vi "SMTP Email Convert SJIS to JIS.vi"(11 "text in":string) -> (3 "text out":string)   [LabVIEW 2012, in "NewNI_SMTPEmail.lvlib"]
doc: "This VI converts SJIS input code to JIS."
uses:
  NewNI_SMTPEmail.lvlib
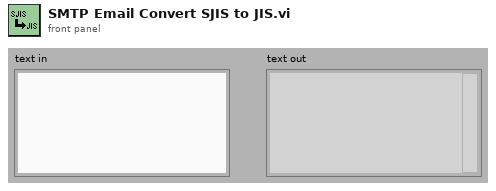
[diagram p1: front panel]
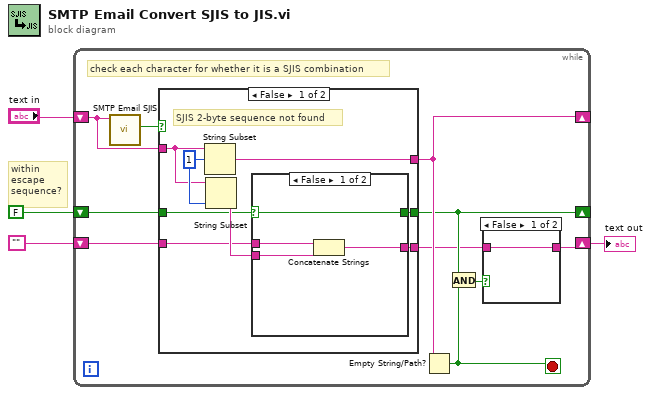
[diagram p0: block diagram]
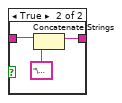
[diagram p2: hidden frame]
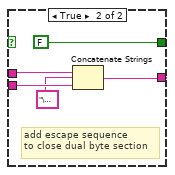
[diagram p3: hidden frame]
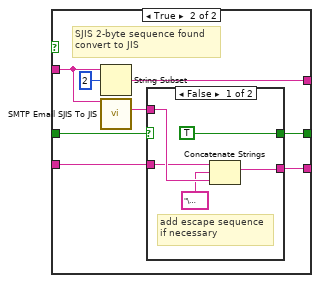
[diagram p4: hidden frame]
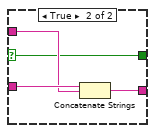
[diagram p5: hidden frame]
diagram:
  # "within\nescape\nsequence?"
  n1 = while {
    shift-right: [w10] -> _
    shift-left: "text in" -> [w13]
    shift-right: [w5] -> w1
    shift-left: "" -> [w12]
    shift-right: [w9] -> _
    shift-left: FALSE -> [w11]
    stop <- w8 stop-if-true
    # "check each character for whether it is a SJIS combination"
    n2 = call "SMTP Email SJIS.vi"("text"=w13) -> ("isSJIS?"=w14:bool)  [unwired: 10 out]
    n3 = case shown="False" w14 {
      tunnel: w13 -> [w24 w39]
      tunnel: [w23 w42] -> w10
      tunnel: w12 -> [w22 w41]
      tunnel: [w20 w40] -> w6
      tunnel: w11 -> [w21 w37]
      tunnel: [w19 w36] -> w9
      frame False {
        w26 = 1 ("offset (0)")
        # "SJIS 2-byte sequence not found"
        n4 = String Subset(string=w24, offset (0)=w26) -> (substring=w23:string)  [unwired: 1 out]
        n5 = String Subset(string=w24, length (rest)=w26) -> (substring=w25:string)  [unwired: 1 out]
        n6 = case shown="False" w21 {
          selector: w21 -> [w27 _]
          tunnel: w25 -> [w30 w35]
          tunnel: w22 -> [w29 w32]
          tunnel: [w28 w34] -> w20
          tunnel: [w27 FALSE] -> w19
          frame False {
            n7 = Concatenate Strings(w29, w30) -> (w28:string)
          }
          frame True {
            # "add escape sequence\nto close dual byte section"
            n8 = Concatenate Strings(w32, "\u001b(J" ("string"), w35) -> (w34:string)
          }
        }
      }
      frame True {
        # "SJIS 2-byte sequence found\nconvert to JIS"
        n9 = String Subset(string=w39, offset (0)=2) -> (substring=w42:string)  [unwired: 1 out]
        n10 = call "SMTP Email SJIS To JIS.vi"("text in"=w39) -> ("text out"=w38:string)  [unwired: 14 out]
        n11 = case shown="False" w37 {
          selector: w37 -> [_ w49]
          tunnel: w41 -> [w45 w52]
          tunnel: [w48 w51] -> w40
          tunnel: w38 -> [w47 w50]
          tunnel: [TRUE w49] -> w36
          frame False {
            # "add escape sequence\nif necessary"
            n12 = Concatenate Strings(w45, "\u001b$B" ("string"), w47) -> (w48:string)
          }
          frame True {
            n13 = Concatenate Strings(w52, w50) -> (w51:string)
          }
        }
      }
    }
    n14 = Empty String/Path?(string/path=w10) -> (empty?=w8:bool)
    n15 = And(x=w9, y=w8) -> (x .and. y?=w7:bool)
    n16 = case shown="False" w7 {
      tunnel: w6 -> [w15 w18]
      tunnel: [w15 w16] -> w5
      frame False {
      }
      frame True {
        n17 = Concatenate Strings(w18, "\u001b(J" ("string")) -> (w16:string)
      }
    }
  }
  "text out" <- w1
